vi "sensor_integration_v2.vi"() -> ()   [LabVIEW 2021]
uses:
  <vilib>/Instr/_visa.llb/VISA Configure Serial Port (Instr).vi
  <vilib>/regexp/Match Regular Expression.xnode
panel:
  out "\"data ok?\" waveform":waveform(i16)(graph)
  out "comm ok?":bool
  out "expected input fmt?":bool
  out "data ok?":bool
  in  "expected \nnum sensors":u32=12
  out "read byte count":u32
  out "error out":errorcluster
  out "flag value ok?":bool[](array[boolean])
  out "temp value ok?":bool[](array[boolean])
  out "flow value ok?":bool[](array[boolean])
  out "high flow flag":bool[](array[boolean])
  out "air in line flag":bool[](array[boolean])
  out "temp data (deg C)":dbl[](array[numeric])
  out "flow rate data (ml/min)":dbl[](array[numeric])
  out "full match?":bool
  out "return byte count":u32
  in  "stop":bool
  out "read buffer":string
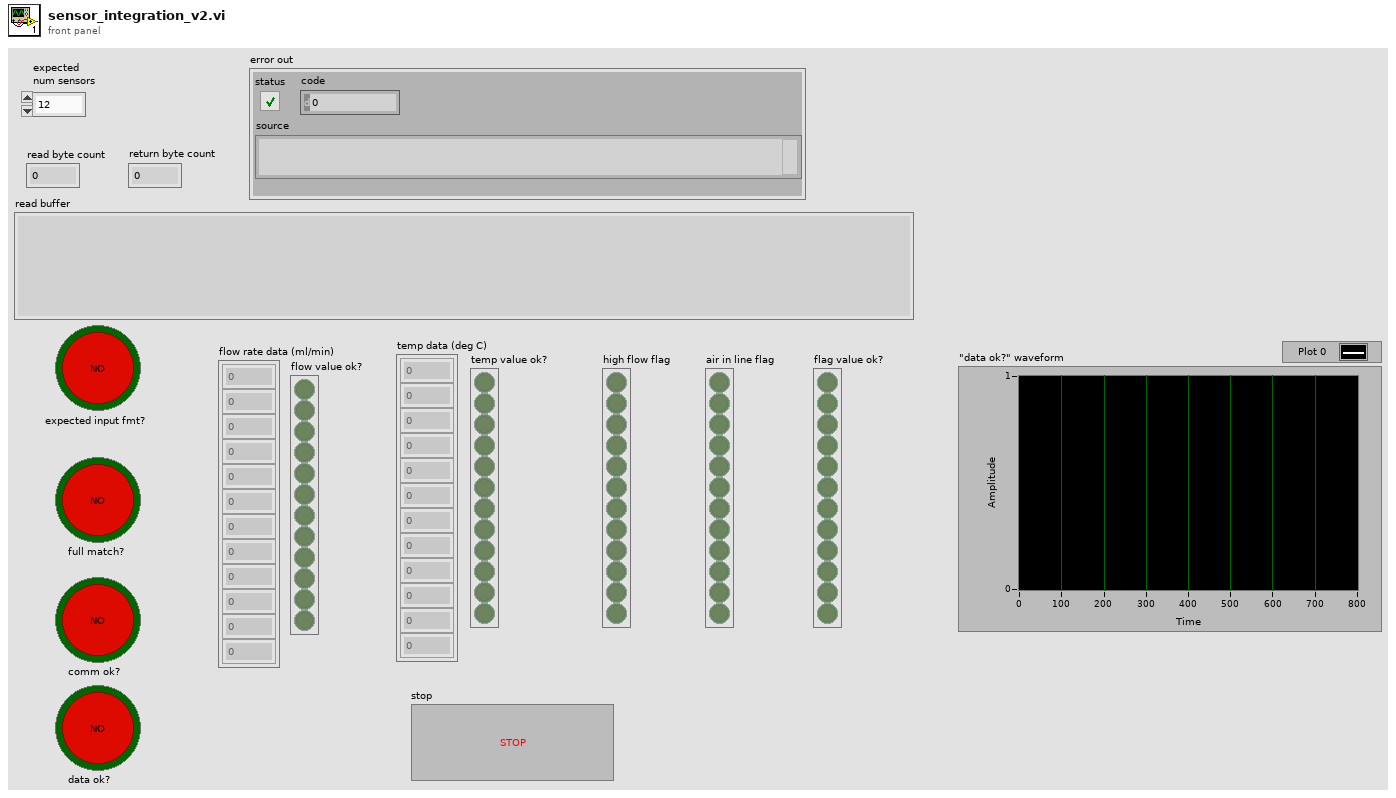
[diagram p1: front panel]
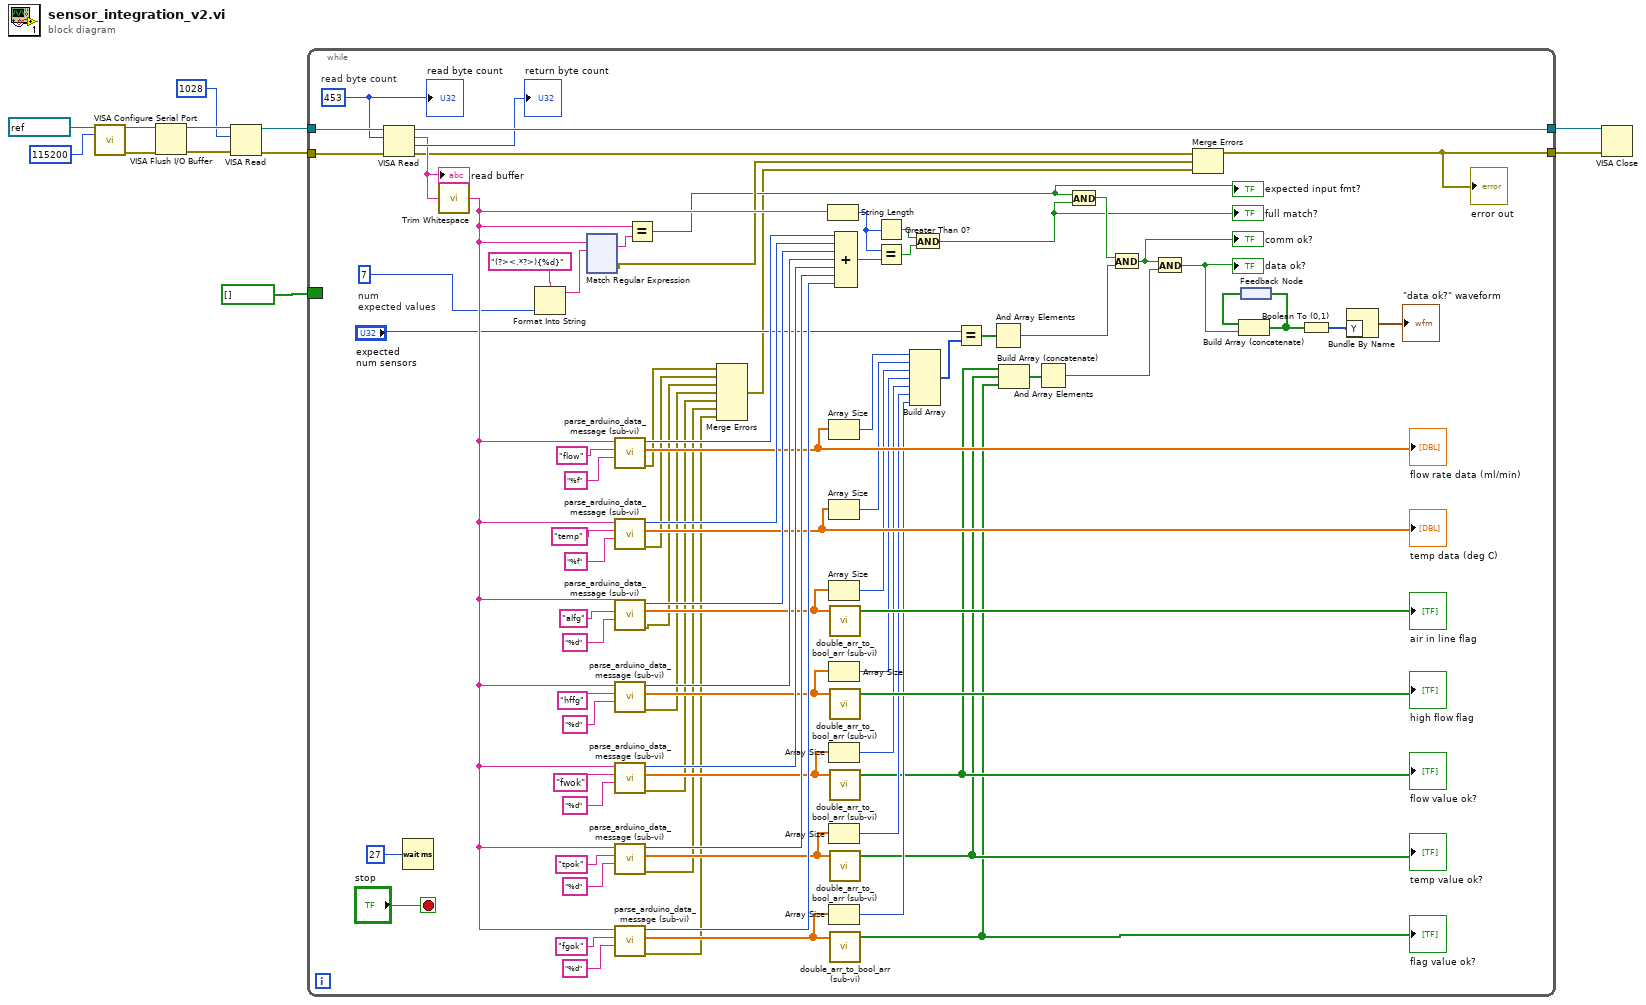
[diagram p0: block diagram]
diagram:
  n1 = call-poly "VISA Configure Serial Port"("VISA resource name"=refnum<visa-resource-name> "COM3", "baud rate (9600)"=u32 115200) -> ("VISA resource name out"=w6:refnum<visa-resource-name>, "error out"=w5:errorcluster)  [unwired: 12 in]
  n2 = VISA Flush I/O Buffer(VISA resource name=w6, error in (no error)=w5) -> (VISA resource name out=w3:refnum<visa-resource-name>, error out=w4:errorcluster)  [unwired: 1 in]
  n3 = VISA Read(VISA resource name=w3, byte count=u32 1028 ("read byte count"), error in (no error)=w4) -> (VISA resource name out=w7:refnum<visa-resource-name>, error out=w8:errorcluster)  [unwired: 2 out]
  n4 = while {
    tunnel: w7 -> [w95]
    tunnel: [w93] -> w12
    tunnel: w8 -> [w90]
    tunnel: [w59] -> w11
    border: bool[] [] -> [_]
    stop <- "stop" stop-if-true
    w39 = 7  # num  expected values
    w61 = u32 453  # read byte count
    n5 = VISA Read(VISA resource name=w95, byte count=w61, error in (no error)=w90) -> (VISA resource name out=w93:refnum<visa-resource-name>, read buffer=w65:string, return count=→"return byte count":u32, error out=w62:errorcluster)
    "read buffer" <- w65
    n6 = Wait (ms)(milliseconds to wait=u32 27) -> ()  [unwired: 1 out]
    n7 = call <vilib>:"Trim Whitespace.vi"("string"=w65) -> ("trimmed string"=w63:string)  [unwired: 1 in]
    n8 = Format Into String(format string="(?><.*?>){%d}" ("input string"), w39) -> (resulting string=w40:string)  [unwired: 2 in, 1 out]
    n9 = xnode "Match Regular Expression"("input string"=w63, "regular expression"=w40) -> ("whole match"=w64:string, "error out"=w60:errorcluster)  [unwired: 4 in, 3 out]
    n10 = call "parse_arduino_data_message (sub-vi).vi"("format string (%f)"="%f" ("input 1"), "data label"="flow" ("input 1"), "input string"=w63) -> ("error out"=w25:errorcluster, "array out"=w52:dbl[], "match length"=w89:i32)  [unwired: 6 in]
    "flow rate data (ml/min)" <- w52
    n11 = call "parse_arduino_data_message (sub-vi).vi"("format string (%f)"="%f" ("input 1"), "data label"="temp" ("input 1"), "input string"=w63) -> ("error out"=w24:errorcluster, "array out"=w58:dbl[], "match length"=w86:i32)  [unwired: 6 in]
    "temp data (deg C)" <- w58
    n12 = call "parse_arduino_data_message (sub-vi).vi"("format string (%f)"="%d" ("input 1"), "data label"="alfg" ("input 1"), "input string"=w63) -> ("error out"=w23:errorcluster, "array out"=w53:dbl[], "match length"=w78:i32)  [unwired: 6 in]
    n13 = call "parse_arduino_data_message (sub-vi).vi"("format string (%f)"="%d" ("input 1"), "data label"="hffg" ("input 1"), "input string"=w63) -> ("error out"=w22:errorcluster, "array out"=w54:dbl[], "match length"=w77:i32)  [unwired: 6 in]
    n14 = call "parse_arduino_data_message (sub-vi).vi"("format string (%f)"="%d" ("input 1"), "data label"="fwok" ("input 1"), "input string"=w63) -> ("error out"=w21:errorcluster, "array out"=w55:dbl[], "match length"=w76:i32)  [unwired: 6 in]
    n15 = call "parse_arduino_data_message (sub-vi).vi"("format string (%f)"="%d" ("input 1"), "data label"="tpok" ("input 1"), "input string"=w63) -> ("error out"=w20:errorcluster, "array out"=w56:dbl[], "match length"=w71:i32)  [unwired: 6 in]
    n16 = call "parse_arduino_data_message (sub-vi).vi"("format string (%f)"="%d" ("input 1"), "data label"="fgok" ("input 1"), "input string"=w63) -> ("error out"=w19:errorcluster, "array out"=w57:dbl[], "match length"=w66:i32)  [unwired: 6 in]
    n17 = Equal?(x=w63, y=w64) -> (x = y?=w31:bool)
    "expected input fmt?" <- w31
    n18 = Merge Errors(w25, w24, w23, w22, w21, w20, w19) -> (w18:errorcluster)
    n19 = String Length(string=w63) -> (length=w26:i32)
    n20 = Array Size(array=w52) -> (size(s)=w51:i32)
    n21 = Array Size(array=w58) -> (size(s)=w50:i32)
    n22 = Array Size(array=w53) -> (size(s)=w49:i32)
    n23 = Array Size(array=w54) -> (size(s)=w48:i32)
    n24 = Array Size(array=w55) -> (size(s)=w47:i32)
    n25 = Array Size(array=w56) -> (size(s)=w46:i32)
    n26 = Array Size(array=w57) -> (size(s)=w45:i32)
    n27 = call "double_arr_to_bool_arr (sub-vi).vi"("double array"=w53) -> ("bool array"=→"air in line flag":bool[])  [unwired: 4 in]
    n28 = call "double_arr_to_bool_arr (sub-vi).vi"("double array"=w54) -> ("bool array"=→"high flow flag":bool[])  [unwired: 4 in]
    n29 = call "double_arr_to_bool_arr (sub-vi).vi"("double array"=w55) -> ("bool array"=w38:bool[])  [unwired: 4 in]
    "flow value ok?" <- w38
    n30 = call "double_arr_to_bool_arr (sub-vi).vi"("double array"=w56) -> ("bool array"=w37:bool[])  [unwired: 4 in]
    "temp value ok?" <- w37
    n31 = call "double_arr_to_bool_arr (sub-vi).vi"("double array"=w57) -> ("bool array"=w36:bool[])  [unwired: 4 in]
    "flag value ok?" <- w36
    n32 = Compound Arithmetic op=ADD(w89, w86, w78, w77, w76, w71, w66) -> (w85:i32)
    n33 = Greater Than 0?(x=w26) -> (x > 0?=w27:bool)
    n34 = Equal?(x=w26, y=w85) -> (x = y?=w29:bool)
    n35 = Build Array(w51, w50, w49, w48, w47, w46, w45) -> (w44:i32[])
    n36 = And(x=w27, y=w29) -> (x .and. y?=w28:bool)
    "full match?" <- w28
    n37 = Equal?(x="expected \nnum sensors", y=w44) -> (x = y?=w43:bool[])
    n38 = And Array Elements(Boolean array=w43) -> (logical AND=w41:bool)
    n39 = Build Array (concatenate)(w38, w37, w36) -> (w35:bool[])
    n40 = And Array Elements(Boolean array=w35) -> (logical AND=w34:bool)
    n41 = And(x=w31, y=w28) -> (x .and. y?=w42:bool)
    n42 = And(x=w42, y=w41) -> (x .and. y?=w32:bool)
    "comm ok?" <- w32
    n43 = And(x=w32, y=w34) -> (x .and. y?=w17:bool)
    "data ok?" <- w17
    n44 = Merge Errors(w62, w60, w18) -> (w59:errorcluster)
    "error out" <- w59
    n45 = feedback #1() -> (w16:bool[])
    n46 = Build Array (concatenate)(w16, w17) -> (w15:bool[])
    n47 = feedback-in #1(w15) -> ()
    n48 = Boolean To (0,1)(Boolean=w15) -> (0, 1=w14:i16[])
    n49 = Bundle By Name("Y"=w14) -> (→"\"data ok?\" waveform":waveform(i16))  [unwired: 1 in]
    "read byte count" <- w61
  }
  n50 = VISA Close(VISA resource name=w12, error in (no error)=w11) -> ()  [unwired: 1 out]
